vi "RichToFlatni_measurementlink_discovery_v1_EnumerateServicesRequest.vi"(5 "OutputClusterType":T1, 11 "InputCluster":T2) -> (3 "OutputCluster":T1)   [LabVIEW 2020, in "ni.measurementlink.discovery.v1.lvlib"]
uses:
  ni.measurementlink.discovery.v1.lvlib
  ni_measurementlink_discovery_v1_EnumerateServicesRequest_Flat.ctl
  ni_measurementlink_discovery_v1_EnumerateServicesRequest.ctl
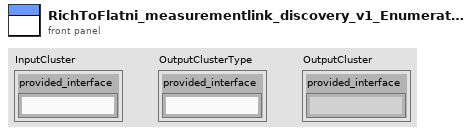
[diagram p1: front panel]
types:
  T1 = typedef "ni.measurementlink.discovery.v1.lvlib/ni_measurementlink_discovery_v1_EnumerateServicesRequest_Flat.ctl" = cluster{"provided_interface":string}
  T2 = typedef "ni.measurementlink.discovery.v1.lvlib/ni_measurementlink_discovery_v1_EnumerateServicesRequest.ctl" = cluster{"provided_interface":string}
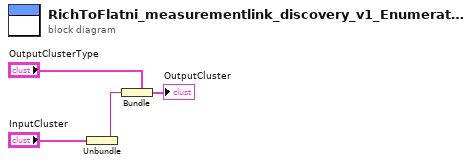
[diagram p0: block diagram]
diagram:
  n1 = Unbundle "Unbundle"("InputCluster") -> ("provided_interface"=w1:string)
  n2 = Bundle "Bundle"(cluster="OutputClusterType", "provided_interface"=w1) -> (→"OutputCluster":T1)
